vi "AlazarGetSystemHandle.vi"(2 "error in (no error)":errorcluster, 3 "System ID":u32) -> (0 "error out":errorcluster, 1 "Handle":u64)   [LabVIEW 2018]
doc: "Return the handle of the master board in the specified board system."
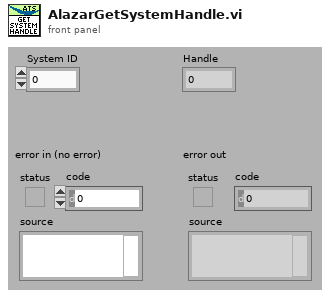
[diagram p1: front panel]
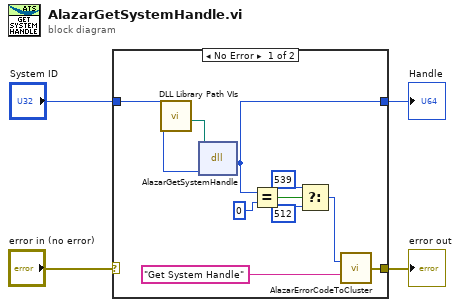
[diagram p0: block diagram]
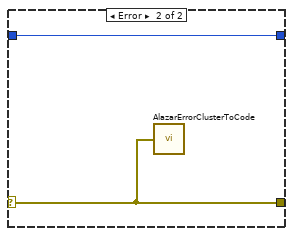
[diagram p2: hidden frame]
diagram:
  n1 = case shown="No Error" "error in (no error)" {
    selector: "error in (no error)" -> [_ w16]
    tunnel: [w12 w16] -> w3
    tunnel: "System ID" -> [w14 w15]
    tunnel: [w6 w15] -> w1
    frame No Error {
      n2 = call "DLL Library Path VIs.vi"() -> ("Alazar"=w5:path)  [unwired: 9 in, 2 out]
      n3 = dll-call lib="C:/Project/SerialSectOCT - FFT GPU/SerialSectOCT/Labview Software/DLL/ATSApi.dll" fn="AlazarGetSystemHandle"(path in=w5, "systemId"=w14) -> ("return type"=w6:u64)  [unwired: 3 in, 2 out]
      n4 = Equal?(x=w6, y=u64 0) -> (x = y?=w10:bool)
      n5 = Select(t=u32 539, s=w10, f=u32 512) -> (s? t:f=w7:u32)
      n6 = call "AlazarErrorCodeToCluster.vi"("Message"="Get System Handle", "Error Code"=w7) -> ("error out"=w12:errorcluster)
    }
    frame Error {
      n7 = call "AlazarErrorClusterToCode.vi"("error in (no error)"=w16) -> ()  [unwired: 1 out]
    }
  }
  "Handle" <- w1
  "error out" <- w3
